vi "init buffer.vi"(8 "error in (no error)":errorcluster, 11 "Data Buffer in":refnum<class "Data Buffer.lvclass">) -> (0 "error out":errorcluster, 3 "Data Buffer out":refnum<class "Data Buffer.lvclass">)   [LabVIEW 2022 SP3, in "Data Buffer.lvclass"]
uses:
  Data Buffer.lvclass
  Data Buffer.lvclass/Data Buffer.ctl
  CC Data buffer Template.vi
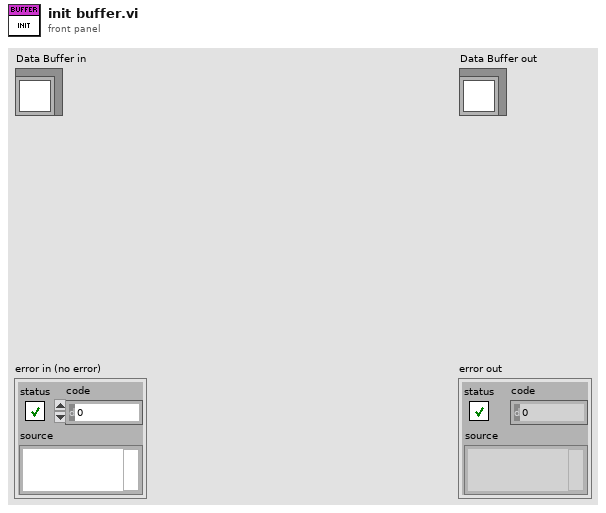
[diagram p1: front panel]
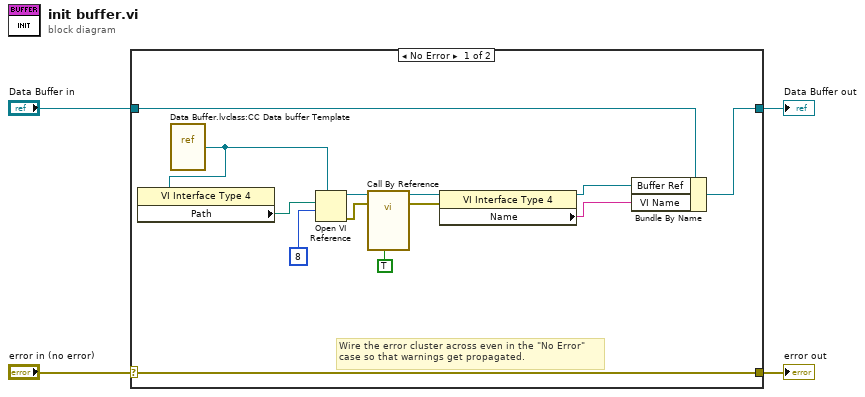
[diagram p0: block diagram]
diagram:
  n1 = case shown="No Error" "error in (no error)" {
    selector: "error in (no error)" -> [w17 w19]
    tunnel: [w17 w19] -> w3
    tunnel: [w10 w18] -> w1
    tunnel: "Data Buffer in" -> [w9 w18]
    frame No Error {
      # "Wire the error cluster across even in the \"No Error\"\ncase so that warnings get propagated."
      n2 = vi-ref "Data Buffer.lvclass:CC Data buffer Template.vi"() -> (w6:refnum<vi>)
      n3 = property class="VI Interface Type 4"(reference=w6) -> ("Path"=w5:path)  [unwired: 1 in, 2 out]
      n4 = Open VI Reference(type specifier VI Refnum (for type only)=w6, vi path=w5, options=8) -> (vi reference=w16:refnum<vi>, error out=w15:errorcluster)  [unwired: 3 in]
      n5 = call-by-ref "?"(reference=w16, error in=w15, "Clear"=TRUE) -> (reference out=w14:refnum<vi>, error out=w13:errorcluster)  [unwired: 9 in, 2 out]
      n6 = property class="VI Interface Type 4"(reference=w14, error in=w13) -> (reference out=w11:refnum<vi>, "Name"=w8:string)  [unwired: 1 out]
      n7 = Bundle By Name(cluster=w9, "Buffer Ref"=w11, "VI Name"=w8) -> (w10:refnum<class "Data Buffer.lvclass">)
    }
    frame Error {
    }
  }
  "error out" <- w3
  "Data Buffer out" <- w1
